vi "Application_CreateTempVICallBat.vi"(7 "TemporaryBatLocation":T1 items=["User Home"=0, "User Desktop"=1, "User Documents"=2, "User Application Data"=3, "User Preferences"=4, "User Temporary"=5, "Public Documents"=6, "Public Application Data"=7, "Public Preferences"=8, "Public Cache"=13, "System Core Libraries"=9, "System Installed Libraries"=10, "Application Files"=11, "Boot Volume Root"=12], 8 "error in":errorcluster, 11 "Project Name":string="BioReactor.lvproj") -> (0 "error IO":errorcluster)   [LabVIEW 2016]
doc: "Creates a windows .bat file with a time delay which is going to restart the project.\n\nAndreas Elmiger, 16.01.2017"
uses:
  <vilib>/Utility/sysdir.llb/System Directory Type.ctl
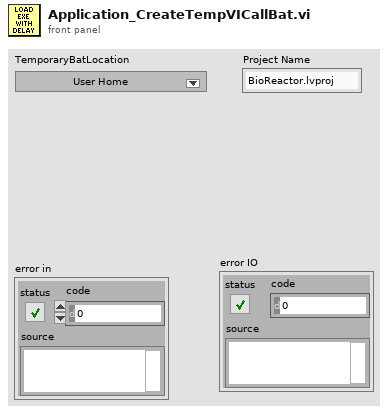
[diagram p1: front panel]
types:
  T1 = typedef "System Directory Type.ctl" = i32
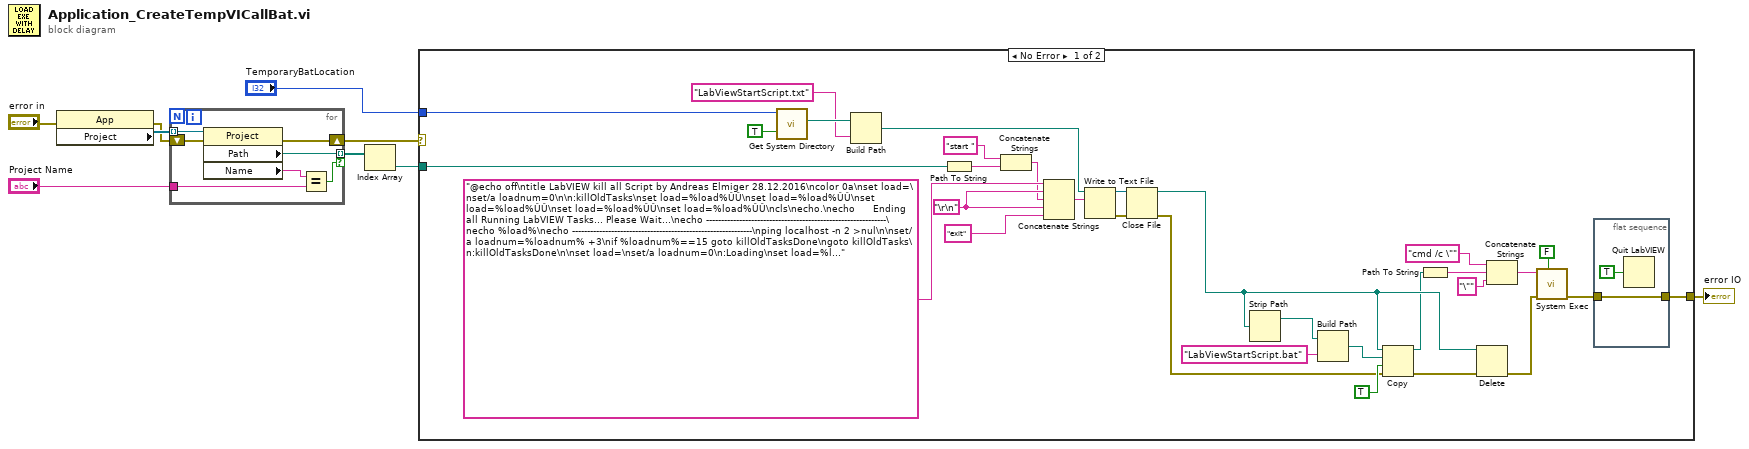
[diagram p0: block diagram]
diagram:
  n1 = property class="App"(error in="error in") -> (error out=w2:errorcluster, "Project"=w7:refnum<vi>[])  [unwired: 1 in, 1 out]
  n2 = for {
    tunnel: w7 -> [w16] mode=indexing
    tunnel: [w15] -> w5 mode=indexing if=w12
    tunnel: "Project Name" -> [w13]
    shift-right: [w10] -> w1
    shift-left: w2 -> [w11]
    n3 = property class="Project"(reference=w16, error in=w11) -> (error out=w10:errorcluster, "Path"=w15:path, "Name"=w14:string)  [unwired: 1 out]
    n4 = Equal?(x=w14, y=w13) -> (x = y?=w12:bool)
  }
  n5 = Index Array(array=w5) -> (element=w4:path)  [unwired: 1 in]
  n6 = case shown="No Error" w1 {
    selector: w1 -> [_ w50]
    tunnel: "TemporaryBatLocation" -> [w47 _]
    tunnel: w4 -> [w27 _]
    tunnel: [w17 w50] -> w8
    frame No Error {
      w29 = "\r\n"
      n7 = call <vilib>:"Get System Directory.vi"("create directory if not found? (F)"=TRUE, "system directory type"=w47) -> ("system directory"=w46:path)  [unwired: 9 in]
      n8 = Build Path(base path=w46, name or relative path="LabViewStartScript.txt" ("prompt (Choose or enter file path)")) -> (appended path=w39:path)
      n9 = Path To String(path=w27) -> (string=w26:string)
      n10 = Concatenate Strings("start " ("string"), w26) -> (w24:string)
      n11 = Concatenate Strings("@echo off\ntitle LabVIEW kill all Script by Andreas Elmiger 28.12.2016\ncolor 0a\nset load=\nset/a loadnum=0\n\n:killOldTasks\nset load=%load%ÛÛ\nset load=%load%ÛÛ\nset load=%load%ÛÛ\nset load=%load%ÛÛ\nset load=%load%ÛÛ\ncls\necho.\necho      Ending all Running LabVIEW Tasks... Please Wait...\necho ------------------------------------------------------------\necho %load%\necho ------------------------------------------------------------\nping localhost -n 2 >nul\n\nset/a loadnum=%loadnum% +3\nif %loadnum%==15 goto killOldTasksDone\ngoto killOldTasks\n:killOldTasksDone\n\nset load=\nset/a loadnum=0\n:Loading\nset load=%load%ÛÛ\nset load=%load%ÛÛ\nset load=%load%ÛÛ\nset load=%load%ÛÛ\nset load=%load%ÛÛ\ncls\necho.\necho         Loading LabVIEW Software... Please Wait...\necho ------------------------------------------------------------\necho %load%\necho ------------------------------------------------------------\nping localhost -n 2 >nul\n\nset/a loadnum=%loadnum% +3\nif %loadnum%==15 goto Done\n\ngoto Loading\n:Done" ("text"), w29, w24, w29, "exit" ("string")) -> (w23:string)
      n12 = Write to Text File(file (use dialog)=w39, text=w23) -> (refnum out=w44:refnum<file>, error out=w22:errorcluster)  [unwired: 2 in, 1 out]
      n13 = Close File(refnum=w44, error in=w22) -> (path=w33:path, error out=w21:errorcluster)
      n14 = Strip Path(path=w33) -> (stripped path=w37:path)  [unwired: 1 out]
      n15 = Build Path(base path=w37, name or relative path="LabViewStartScript.bat") -> (appended path=w36:path)
      n16 = Copy(8:w21, 9:TRUE ("overwrite (F)"), 10:w36, 11:w33) -> (0:w34:errorcluster, 3:w32:path)  [unwired: 1 in, 1 out]
      n17 = Path To String(path=w32) -> (string=w41:string)
      n18 = Delete(path (use dialog)=w33, error in=w34) -> (error out=w19:errorcluster)  [unwired: 3 in, 2 out]
      n19 = Concatenate Strings("cmd /c \"" ("command line"), w41, "\"" ("string")) -> (w42:string)
      n20 = call <vilib>:"System Exec.vi"("wait until completion? (T)"=FALSE, "error in (no error)"=w19, "command line"=w42) -> ("error out"=w18:errorcluster)  [unwired: 5 in, 3 out]
      n21 = flat-sequence {
        tunnel: w18 -> [w48]
        tunnel: [w48] -> w17
        frame #0 {
          n22 = Quit LabVIEW(quit? (T)=TRUE) -> ()
        }
      }
    }
    frame Error {
    }
  }
  "error IO" <- w8
